vi "Status Log FGV.vi"(7 "Action":T1=enum."Show Status File", 8 "error in":errorcluster, 10 "Status":string) -> (0 "error out":errorcluster)   [LabVIEW 2015]
uses:
  Status Log.ctl
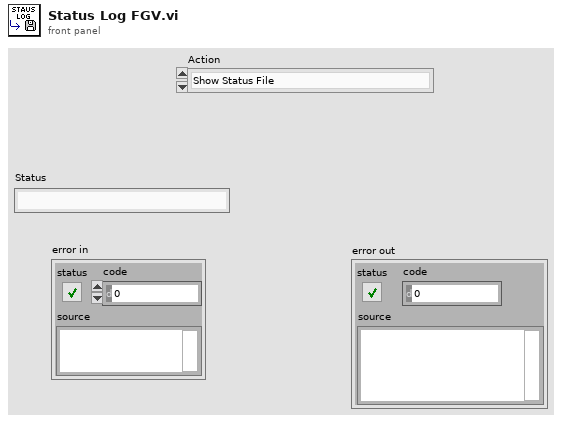
[diagram p1: front panel]
types:
  T1 = typedef "Status Log.ctl" = enum16{"Close file", "Open Status file", "Add Status", "Show Status File"}
  T2 = enum16{"open", "replace", "create", "open or create", "replace or create", "replace or create with confirmation"}
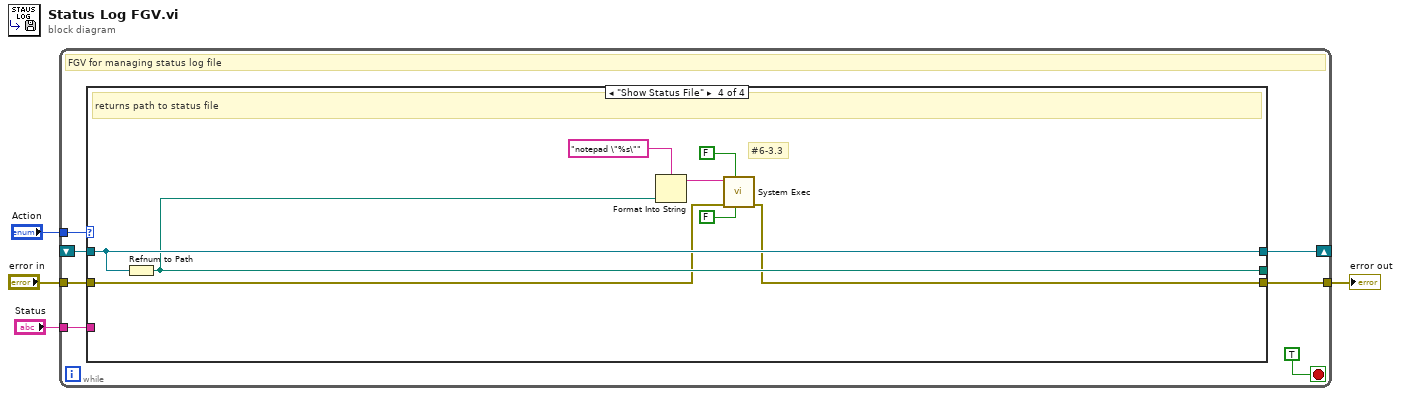
[diagram p0: block diagram]
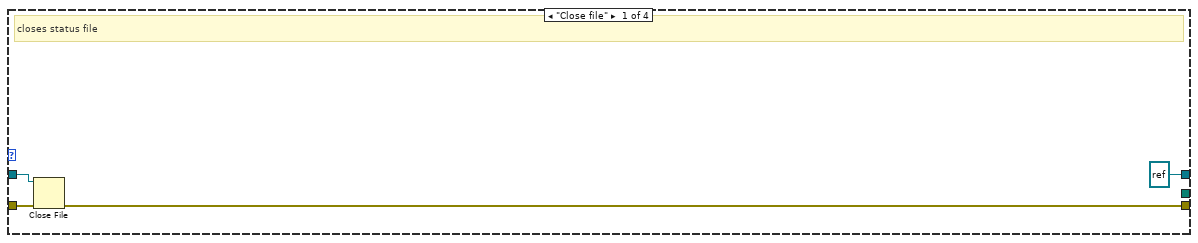
[diagram p2: hidden frame]
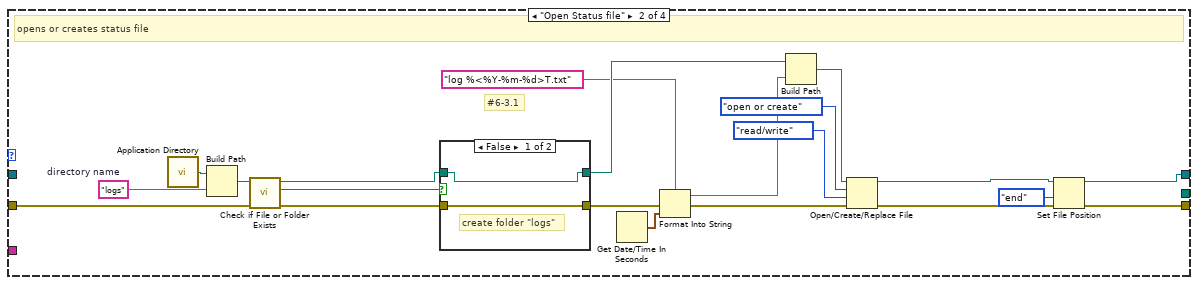
[diagram p3: hidden frame]
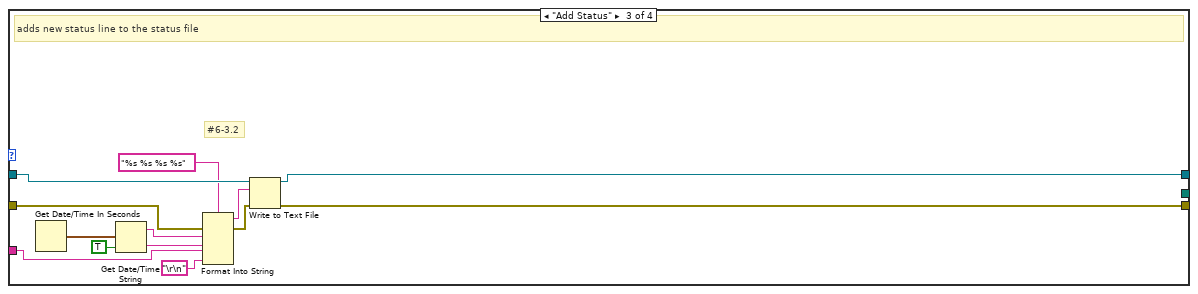
[diagram p5: hidden frame]
diagram:
  n1 = while {
    tunnel: "Action" -> [w10]
    tunnel: "Status" -> [w9]
    tunnel: [w8] -> w2
    tunnel: "error in" -> [w7]
    shift-right: [w5] -> _
    shift-left: _ -> [w6]
    stop <- TRUE stop-if-true
    # "FGV for managing status log file"
    n2 = case shown="\"Show Status File\"" w10 {
      tunnel: w9 -> [_ _ w44 _]
      tunnel: [w14 w28 w53 w57] -> w8
      tunnel: w7 -> [w15 w21 w45 w58]
      tunnel: [refnum<file> refnum ("refnum out") w27 w52 w61] -> w5
      tunnel: w6 -> [w13 _ w51 w61]
      tunnel: [_ _ _ w59] -> _
      frame "Close file" {
        # "closes status file"
        n3 = Close File(refnum=w13, error in=w15) -> (error out=w14:errorcluster)  [unwired: 1 out]
      }
      frame "Open Status file" {
        w17 = "logs"  # directory name
        # "#6-3.1"
        # "opens or creates status file"
        n4 = call <vilib>:"Application Directory.vi"() -> ("Application Directory"=w36:path)
        n5 = Build Path(base path=w36, name or relative path=w17) -> (appended path=w26:path)
        n6 = call <vilib>:"Check if File or Folder Exists.vi"("error in (no error)"=w21, "path"=w26) -> ("error out"=w22:errorcluster, "file or folder exists?"=w25:bool, "dup path"=w24:path)  [unwired: 7 in]
        n7 = case shown="False" w25 {
          tunnel: w24 -> [w38 w40]
          tunnel: [w38 w40] -> w23
          tunnel: w22 -> [w37 w39]
          tunnel: [w37 w39] -> w20
          frame False {
            # "create folder \"logs\""
          }
          frame True {
          }
        }
        n8 = Get Date/Time In Seconds() -> (seconds since 1Jan1904=w35:timestamp)
        n9 = Format Into String "Format Into String"(format string="log %<%Y-%m-%d>T.txt", error in=w20, w35) -> (resulting string=w33:string, error out=w34:errorcluster)  [unwired: 1 in]
        n10 = Build Path(base path=w23, name or relative path=w33) -> (appended path=w32:path)
        n11 = Open/Create/Replace File(file path (use dialog)=w32, error in=w34, operation (0:open)=T2."open or create", access (0:read/write)=enum16{"read/write", "read-only", "write-only"}."read/write") -> (refnum out=w29:refnum<file>, error out=w30:errorcluster)  [unwired: 2 in, 1 out]
        n12 = Set File Position(refnum=w29, from (0:start)=enum16{"start", "end", "current"}."end", error in=w30) -> (refnum out=w27:refnum<file>, error out=w28:errorcluster)  [unwired: 1 in]
      }
      frame "Add Status" {
        # "#6-3.2"
        # "adds new status line to the status file"
        n13 = Get Date/Time In Seconds() -> (seconds since 1Jan1904=w49:timestamp)
        n14 = Get Date/Time String(seconds (now)=w49, want seconds? (F)=TRUE) -> (date string=w48:string, time string=w47:string)  [unwired: 1 in]
        n15 = Format Into String(format string="%s %s %s %s", error in=w45, w48, w47, w44, "\r\n") -> (resulting string=w41:string, error out=w43:errorcluster)  [unwired: 1 in]
        n16 = Write to Text File(file (use dialog)=w51, text=w41, error in=w43) -> (refnum out=w52:refnum<file>, error out=w53:errorcluster)  [unwired: 1 in, 1 out]
      }
      frame "Show Status File" {
        # "#6-3.3"
        # "returns path to status file"
        n17 = Refnum to Path(1:w61) -> (0:w59:path)
        n18 = Format Into String(format string="notepad \"%s\"", w59) -> (resulting string=w60:string)  [unwired: 2 in, 1 out]
        n19 = call <vilib>:"System Exec.vi"("run minimized? (F)"=FALSE, "wait until completion? (T)"=FALSE, "error in (no error)"=w58, "command line"=w60) -> ("error out"=w57:errorcluster)  [unwired: 4 in, 3 out]
      }
    }
  }
  "error out" <- w2
